vi "CTR_XML-expand.vi"(8 "error in":errorcluster, 9 "XML file path":path, 10 "channel Definitions":T1, 11 "DOM document in":refnum<k20>) -> (0 "error out":errorcluster={"status"=TRUE, "code"=0, "source"=""}, 3 "DOM document out":refnum<k20>)   [LabVIEW 2024]
uses:
  Control/CTR_channelDefinitions.ctl
  <vilib>/xml/Close Reference(Node).vi
  <vilib>/xml/Load XML File.vi
  <vilib>/Utility/error.llb/Error Cluster From Error Code.vi
  OneDrive - Embry-Riddle Aeronautical University/Admin/Facilities/TC3/TC3 DAC/Code/RTC_PXIe-Code v1_9_0 CODE/Configs/parsedConfigs/DOM document.vi
  <vilib>/ErrorRing/Error Ring.xnode
  <vilib>/xml/NI_XML.lvlib
  <resource>/objmgr/DOMUserDefRef.rc
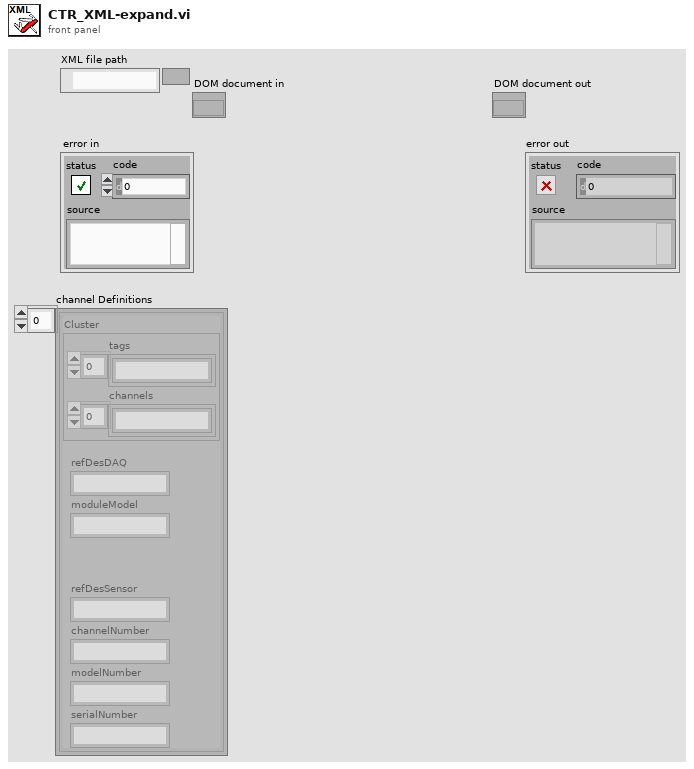
[diagram p1: front panel]
types:
  T1 = typedef "CTR_channelDefinitions.ctl" = cluster{"refDesDAQ":string, "moduleModel":string, "refDesSensor":string, "channelNumber":string, "modelNumber":string, "serialNumber":string, "Cluster":cluster{"tags":string[], "channels":string[]}}[]
  T2 = cluster{"refDesSensor":string, "serialNumber":string, "modelNumber":string, "channelNumber":string}
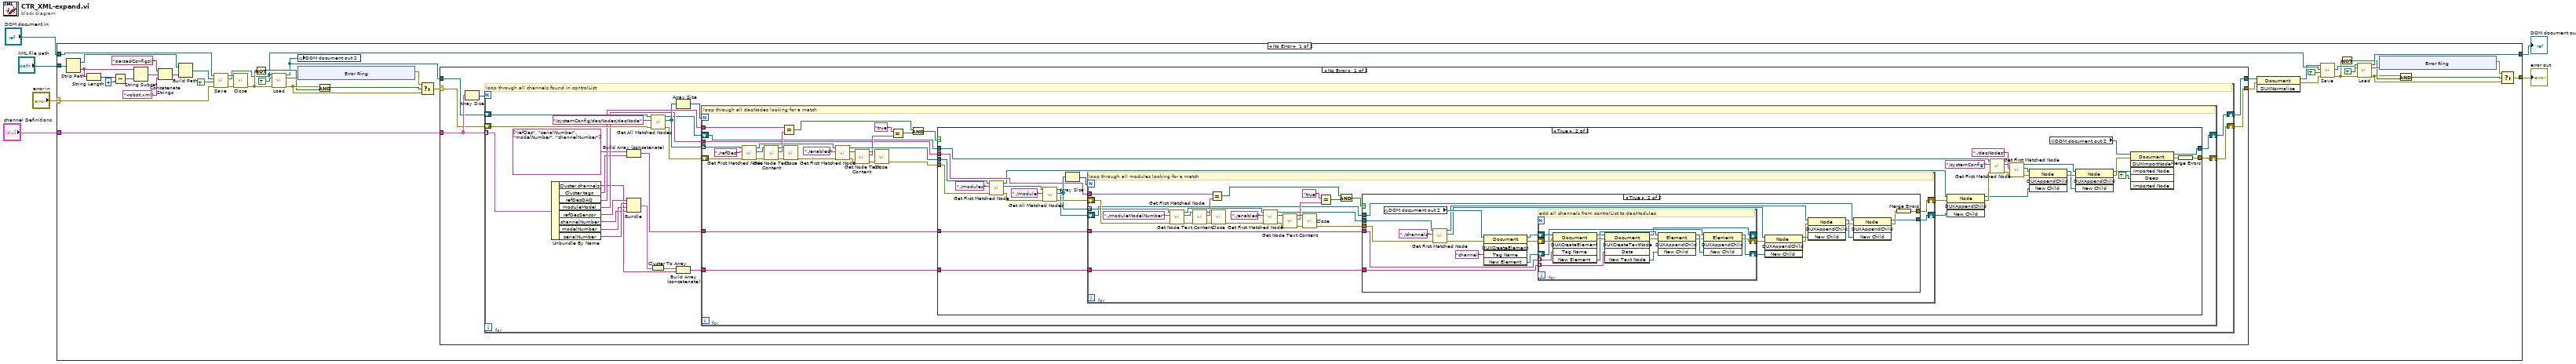
[diagram p0: block diagram]
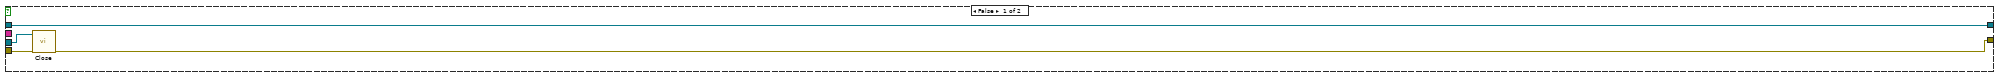
[diagram p2: hidden frame]
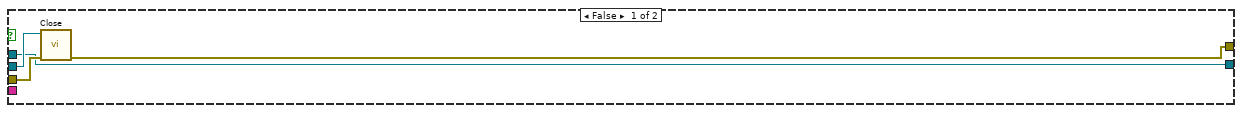
[diagram p3: hidden frame]
diagram:
  n1 = case shown="No Error" "error in" {
    selector: "error in" -> [w36 w233]
    tunnel: [w7 w233] -> w5
    tunnel: [w14 w232] -> w4
    tunnel: "DOM document in" -> [w46 w232]
    tunnel: "channel Definitions" -> [w48 _]
    tunnel: "XML file path" -> [w45 _]
    frame No Error {
      n2 = Strip Path(path=w45) -> (stripped path=w38:path, name=w29:string)
      n3 = String Length(string=w29) -> (length=w44:i32)
      n4 = Subtract(x=w44, y=4) -> (x-y=w28:i32)
      n5 = String Subset(string=w29, length (rest)=w28) -> (substring=w42:string)  [unwired: 1 in]
      n6 = Concatenate Strings("parsedConfigs\\" ("string"), w42, "-robot.xml" ("string")) -> (w39:string)
      n7 = Build Path(base path=w38, name or relative path=w39) -> (appended path=w37:path)
      n8 = call <vilib>:"Save.vi"("error in (no error)"=w36, "overwrite file (True)"=TRUE, "XML file path"=w37, "DOM document in"=w46) -> ("error out"=w35:errorcluster, "XML file path out"=w22:path, "DOM document out"=w34:refnum<k20>)  [unwired: 5 in]
      n9 = call-poly <vilib>:"Close.vi"("error in (no error)"=w35, "node"=w34) -> ("error out"=w27:errorcluster)  [unwired: 7 in]
      n10 = Not(x=w27) -> (.not. x?=w24:bool)
      n11 = call-poly <vilib>:"Load.vi"("path to XML document"=w22, "process namespaces (False)"=TRUE, "error in (no error)"=w27) -> ("DOM document out"=w21:refnum<k20>, "parse errors"=w30:string, "error out"=w26:errorcluster)  [unwired: 10 in]
      n12 = global write "DOM document.vi" "DOM document out 2"(w21) -> ()
      n13 = xnode "Error Ring"("parameter 0"=w30) -> ("error out"=w32:errorcluster)
      n14 = And(x=w26, y=w24) -> (x .and. y?=w25:bool)
      n15 = Select(t=w32, s=w25, f=w26) -> (s? t:f=w31:errorcluster)
      n16 = case shown="No Error" w31 {
        selector: w31 -> [w64 w231]
        tunnel: [w68 w231] -> w20
        tunnel: w48 -> [w66 _]
        tunnel: w21 -> [w65 w230]
        tunnel: [w63 w230] -> w19
        frame No Error {
          n17 = Array Size(array=w66) -> (size(s)=w67:i32)
          n18 = for {
            N: w67 -> [_]
            shift-right: [w82] -> w68
            shift-left: w64 -> [w90]
            tunnel: w66 -> [w88] mode=indexing
            shift-right: [w69] -> w63
            shift-left: w65 -> [w91]
            # "loop through all channels found in controlList"
            n19 = Unbundle By Name(w88) -> ("Cluster.channels"=w71:string[], "Cluster.tags"=w74:string[], "refDesDAQ"=w86:string, "moduleModel"=w83:string, "refDesSensor"=w81:string, "channelNumber"=w78:string, "modelNumber"=w79:string, "serialNumber"=w80:string)
            n20 = Bundle("refDesSensor"=w81, "serialNumber"=w80, "modelNumber"=w79, "channelNumber"=w78) -> (w77:T2)  [unwired: 1 in]
            n21 = Build Array (concatenate)(string[] ["refDes", "serialNumber", "modelNumber", "channelNumber"], w74) -> (w75:string[])
            n22 = Cluster To Array(cluster=w77) -> (array=w73:string[])
            n23 = call <vilib>:"Get All Matched Nodes.vi"("error in (no error)"=w90, "XPath expression"="/systemConfig/daqNodes/daqNode", "node in"=w91) -> ("error out"=w89:errorcluster, "node result array"=w85:refnum<k20>[], "node out"=w70:refnum<k20>)  [unwired: 6 in]
            n24 = Array Size(array=w85) -> (size(s)=w84:i32)
            n25 = Build Array (concatenate)(w73, w71) -> (w72:string[])
            n26 = for {
              N: w84 -> [_]
              tunnel: w85 -> [w115] mode=indexing
              shift-right: [w94] -> w82
              shift-left: w89 -> [w116]
              tunnel: w86 -> [w112]
              tunnel: w83 -> [w97]
              tunnel: w72 -> [w96]
              tunnel: w75 -> [w95]
              shift-right: [w92] -> w69
              shift-left: w70 -> [w93]
              # "loop through all daqNodes looking for a match"
              n27 = call <vilib>:"Get First Matched Node.vi"("error in (no error)"=w116, "XPath expression"="./refDes", "node in"=w115) -> ("error out"=w118:errorcluster, "node result"=w119:refnum<k20>, "node out"=w106:refnum<k20>)  [unwired: 6 in]
              n28 = call <vilib>:"Get Node Text Content.vi"("error in (no error)"=w118, "node in"=w119) -> ("error out"=w117:errorcluster, "node text"=w113:string, "node out"=w120:refnum<k20>)  [unwired: 7 in]
              n29 = Equal?(x=w112, y=w113) -> (x = y?=w110:bool)
              n30 = call-poly <vilib>:"Close.vi"("error in (no error)"=w117, "node"=w120) -> ("error out"=w107:errorcluster)  [unwired: 7 in]
              n31 = call <vilib>:"Get First Matched Node.vi"("error in (no error)"=w107, "XPath expression"="./enabled", "node in"=w106) -> ("error out"=w108:errorcluster, "node result"=w100:refnum<k20>, "node out"=w105:refnum<k20>)  [unwired: 6 in]
              n32 = call <vilib>:"Get Node Text Content.vi"("error in (no error)"=w108, "node in"=w100) -> ("error out"=w109:errorcluster, "node text"=w104:string, "node out"=w101:refnum<k20>)  [unwired: 7 in]
              n33 = call-poly <vilib>:"Close.vi"("error in (no error)"=w109, "node"=w101) -> ("error out"=w98:errorcluster)  [unwired: 7 in]
              n34 = Equal?(x="true", y=w104) -> (x = y?=w102:bool)
              n35 = And(x=w110, y=w102) -> (x .and. y?=w111:bool)
              n36 = case shown="True" w111 {
                tunnel: [w122 w125] -> w94
                tunnel: w98 -> [w124 w149]
                tunnel: w105 -> [w123 w150]
                tunnel: w97 -> [_ w155]
                tunnel: w96 -> [_ w154]
                tunnel: w95 -> [_ w153]
                tunnel: w93 -> [w121 w144]
                tunnel: [w121 w129] -> w92
                frame False {
                  n37 = call-poly <vilib>:"Close.vi"("error in (no error)"=w124, "node"=w123) -> ("error out"=w122:errorcluster)  [unwired: 7 in]
                }
                frame True {
                  n38 = call <vilib>:"Get First Matched Node.vi"("error in (no error)"=w149, "XPath expression"="./modules", "node in"=w150) -> ("error out"=w146:errorcluster, "node result"=w147:refnum<k20>, "node out"=w145:refnum<k20>)  [unwired: 6 in]
                  n39 = call <vilib>:"Get All Matched Nodes.vi"("error in (no error)"=w146, "XPath expression"="./module", "node in"=w147) -> ("error out"=w159:errorcluster, "node result array"=w157:refnum<k20>[], "node out"=w151:refnum<k20>)  [unwired: 6 in]
                  n40 = Array Size(array=w157) -> (size(s)=w156:i32)
                  n41 = for {
                    N: w156 -> [_]
                    shift-right: [w161] -> w152
                    shift-left: w159 -> [w172]
                    tunnel: w157 -> [w171] mode=indexing
                    tunnel: w155 -> [w170]
                    tunnel: w154 -> [w164]
                    tunnel: w153 -> [w163]
                    shift-right: [w160] -> w132
                    shift-left: w151 -> [w162]
                    # "loop through all modules looking for a match"
                    n42 = call <vilib>:"Get First Matched Node.vi"("error in (no error)"=w172, "XPath expression"="./moduleModelNumber", "node in"=w171) -> ("error out"=w178:errorcluster, "node result"=w177:refnum<k20>, "node out"=w184:refnum<k20>)  [unwired: 6 in]
                    n43 = call <vilib>:"Get Node Text Content.vi"("error in (no error)"=w178, "node in"=w177) -> ("error out"=w179:errorcluster, "node text"=w180:string, "node out"=w176:refnum<k20>)  [unwired: 7 in]
                    n44 = Equal?(x=w170, y=w180) -> (x = y?=w168:bool)
                    n45 = call-poly <vilib>:"Close.vi"("error in (no error)"=w179, "node"=w176) -> ("error out"=w183:errorcluster)  [unwired: 7 in]
                    n46 = call <vilib>:"Get First Matched Node.vi"("error in (no error)"=w183, "XPath expression"="./enabled", "node in"=w184) -> ("error out"=w182:errorcluster, "node result"=w187:refnum<k20>, "node out"=w165:refnum<k20>)  [unwired: 6 in]
                    n47 = call <vilib>:"Get Node Text Content.vi"("error in (no error)"=w182, "node in"=w187) -> ("error out"=w181:errorcluster, "node text"=w185:string, "node out"=w186:refnum<k20>)  [unwired: 7 in]
                    n48 = call-poly <vilib>:"Close.vi"("error in (no error)"=w181, "node"=w186) -> ("error out"=w166:errorcluster)  [unwired: 7 in]
                    n49 = Equal?(x="true", y=w185) -> (x = y?=w169:bool)
                    n50 = And(x=w168, y=w169) -> (x .and. y?=w167:bool)
                    n51 = case shown="True" w167 {
                      tunnel: w166 -> [w191 w212]
                      tunnel: [w190 w200] -> w161
                      tunnel: w165 -> [w189 w213]
                      tunnel: w164 -> [_ w210]
                      tunnel: w163 -> [_ w208]
                      tunnel: w162 -> [w188 w198]
                      tunnel: [w188 w194] -> w160
                      frame False {
                        n52 = call-poly <vilib>:"Close.vi"("error in (no error)"=w191, "node"=w189) -> ("error out"=w190:errorcluster)  [unwired: 7 in]
                      }
                      frame True {
                        n53 = global read "DOM document.vi" "DOM document out 2"() -> (w205:refnum<k20>)
                        n54 = call <vilib>:"Get First Matched Node.vi"("error in (no error)"=w212, "XPath expression"="./channels", "node in"=w213) -> ("error out"=w197:errorcluster, "node result"=w203:refnum<k20>, "node out"=w202:refnum<k20>)  [unwired: 6 in]
                        n55 = invoke class="Document" method="DUXCreateElement"(reference=w205, error in=w197, "Tag Name"="channel") -> (reference out=w206:refnum<k20>, error out=w209:errorcluster, "New Element"=w207:refnum<k20>)  [unwired: 2 in, 2 out]
                        n56 = for {
                          tunnel: w210 -> [w224] mode=indexing
                          shift-right: [w218] -> w192
                          shift-left: w209 -> [w228]
                          tunnel: w208 -> [w227] mode=indexing
                          shift-right: [w219] -> w193
                          shift-left: w207 -> [w220]
                          shift-right: [w217] -> _
                          shift-left: w206 -> [w229]
                          # "add all channels from controlList to daqModules"
                          n57 = invoke class="Document" method="DUXCreateElement"(reference=w229, error in=w228, "Tag Name"=w227) -> (reference out=w226:refnum<k20>, error out=w225:errorcluster, "New Element"=w221:refnum<k20>)  [unwired: 2 in, 2 out]
                          n58 = invoke class="Document" method="DUXCreateTextNode"(reference=w226, error in=w225, "Data"=w224) -> (reference out=w217:refnum<k20>, error out=w223:errorcluster, "New Text Node"=w222:refnum<k20>)  [unwired: 2 in, 2 out]
                          n59 = invoke class="Element" method="DUXAppendChild"(reference=w221, error in=w223, "New Child"=w222) -> (reference out=w216:refnum<k20>, error out=w215:errorcluster)  [unwired: 1 in, 2 out]
                          n60 = invoke class="Element" method="DUXAppendChild"(reference=w220, error in=w215, "New Child"=w216) -> (reference out=w219:refnum<k20>, error out=w218:errorcluster)  [unwired: 1 in, 2 out]
                        }
                        n61 = invoke class="Node" method="DUXAppendChild"(reference=w203, error in=w192, "New Child"=w193) -> (reference out=w195:refnum<k20>, error out=w204:errorcluster)  [unwired: 1 in, 2 out]
                        n62 = invoke class="Node" method="DUXAppendChild"(reference=w202, error in=w204, "New Child"=w195) -> (reference out=w196:refnum<k20>, error out=w201:errorcluster)  [unwired: 1 in, 2 out]
                        n63 = invoke class="Node" method="DUXAppendChild"(reference=w198, error in=w201, "New Child"=w196) -> (reference out=w194:refnum<k20>, error out=w199:errorcluster)  [unwired: 1 in, 2 out]
                        n64 = Merge Errors(w199) -> (w200:errorcluster)
                      }
                    }
                  }
                  n65 = invoke class="Node" method="DUXAppendChild"(reference=w145, error in=w152, "New Child"=w132) -> (reference out=w131:refnum<k20>, error out=w143:errorcluster)  [unwired: 1 in, 2 out]
                  n66 = call <vilib>:"Get First Matched Node.vi"("error in (no error)"=w143, "XPath expression"="/systemConfig", "node in"=w144) -> ("error out"=w142:errorcluster, "node result"=w134:refnum<k20>)  [unwired: 6 in, 1 out]
                  n67 = call <vilib>:"Get First Matched Node.vi"("error in (no error)"=w142, "XPath expression"="./daqNodes", "node in"=w134) -> ("error out"=w139:errorcluster, "node result"=w138:refnum<k20>, "node out"=w135:refnum<k20>)  [unwired: 6 in]
                  n68 = invoke class="Node" method="DUXAppendChild"(reference=w138, error in=w139, "New Child"=w131) -> (reference out=w130:refnum<k20>, error out=w137:errorcluster)  [unwired: 1 in, 2 out]
                  n69 = global read "DOM document.vi" "DOM document out 2"() -> (w127:refnum<k20>)
                  n70 = invoke class="Node" method="DUXAppendChild"(reference=w135, error in=w137, "New Child"=w130) -> (reference out=w128:refnum<k20>, error out=w133:errorcluster)  [unwired: 1 in, 2 out]
                  n71 = invoke class="Document" method="DUXImportNode"(reference=w127, error in=w133, "Imported Node"=w128, "Deep"=TRUE) -> (reference out=w129:refnum<k20>, error out=w136:errorcluster)  [unwired: 2 in, 4 out]
                  n72 = Merge Errors(w136) -> (w125:errorcluster)
                }
              }
            }
          }
        }
        frame Error {
        }
      }
      n73 = invoke class="Document" method="DUXNormalize"(reference=w19, error in=w20) -> (reference out=w18:refnum<k20>, error out=w17:errorcluster)  [unwired: 1 in, 1 out]
      n74 = call <vilib>:"Save.vi"("error in (no error)"=w17, "overwrite file (True)"=TRUE, "XML file path"=w22, "DOM document in"=w18) -> ("error out"=w10:errorcluster, "XML file path out"=w16:path)  [unwired: 5 in, 1 out]
      n75 = Not(x=w10) -> (.not. x?=w12:bool)
      n76 = call-poly <vilib>:"Load.vi"("path to XML document"=w16, "process namespaces (False)"=TRUE, "error in (no error)"=w10) -> ("DOM document out"=w14:refnum<k20>, "parse errors"=w13:string, "error out"=w11:errorcluster)  [unwired: 10 in]
      n77 = xnode "Error Ring"("parameter 0"=w13) -> ("error out"=w8:errorcluster)
      n78 = And(x=w11, y=w12) -> (x .and. y?=w9:bool)
      n79 = Select(t=w8, s=w9, f=w11) -> (s? t:f=w7:errorcluster)
    }
    frame Error {
    }
  }
  "error out" <- w5
  "DOM document out" <- w4
